vi "Get Pin.vi"(0 "NXP in":refnum<class "NXP.lvclass">, 5 "VISA resource name":refnum<visa-resource-name>, 9 "Pin":u8, 11 "error in (no error)":errorcluster) -> (4 "NXP out":refnum<class "NXP.lvclass">, 6 "VISA resource name 2":refnum<visa-resource-name>, 8 "Boolean":bool, 10 "Response":string, 15 "error out":errorcluster)   [LabVIEW 2020, in "NXP.lvclass"]
doc: "Get Pin de NXP\nUsando los parámetros establecidos en el Vi del papá, este VI obtiene uno de los 4 pines configurados en NXP, si esta presionado en la tarjeta me marca un true y si no me marca un false"
uses:
  NXP.lvclass
  7e851a0d-8085-469e-89df-d31a43da1971.vi
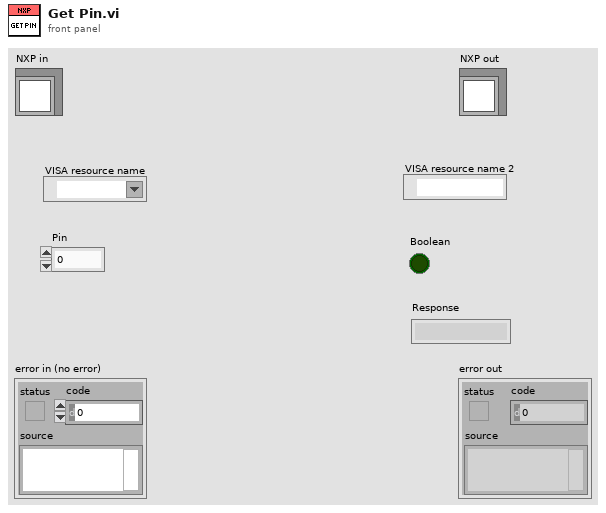
[diagram p1: front panel]
types:
  T1 = enum16{"Write", "Read", "Config", "Reset", "Close"}
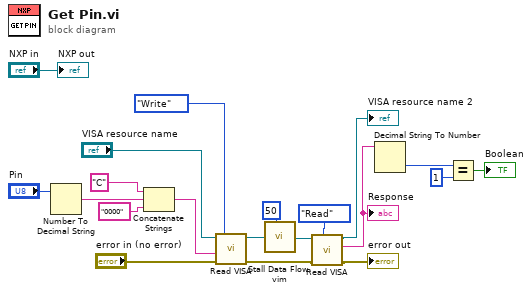
[diagram p0: block diagram]
diagram:
  n1 = Number To Decimal String(number="Pin") -> (decimal integer string=w18:string)  [unwired: 1 in]
  n2 = Concatenate Strings("C" ("string"), w18, "0000" ("string")) -> (w9:string)
  n3 = call "Read VISA.vi"("Opciones"=T1."Write", "error in (no error)"="error in (no error)", "Write"=w9, "VISA com port"="VISA resource name") -> ("error out"=w5:errorcluster, "VISA com port 2"=w7:refnum<visa-resource-name>)  [unwired: 5 in, 1 out]
  n4 = call "Stall Data Flow.vim"("value in"=w7, "milliseconds to wait"=u32 50) -> ("value out"=w4:refnum<visa-resource-name>)  [unwired: 1 out]
  n5 = call "Read VISA.vi"("Opciones"=T1."Read", "error in (no error)"=w5, "VISA com port"=w4) -> ("error out"=→"error out":errorcluster, "Read"=w1:string, "VISA com port 2"=→"VISA resource name 2":refnum<visa-resource-name>)  [unwired: 6 in]
  "Response" <- w1
  n6 = Decimal String To Number(string=w1) -> (number=w15:i32)  [unwired: 2 in, 1 out]
  n7 = Equal?(x=w15, y=1) -> (x = y?=→"Boolean":bool)
  "NXP out" <- "NXP in"
